vi "ImageGUI.vi"() -> ()   [LabVIEW 2017]
uses:
  <vilib>/Utility/miscctls.llb/LVPoint32TypeDef.ctl
  <vilib>/userdefined/High Color/IMAQdx.ctl
  <vilib>/vision/driver/NI_Vision_Acquisition_Software.lvlib
  <vilib>/vision/NI_Vision_Development_Module.lvlib
panel:
  out "Standard Variation":sgl
  out "SnapshotObjects":T1(array[cluster]) {"Aspect Ratio" format="%.2f"; "Orientation" format="%.2f"; "Area" format="%.2f"; "Object Center"."Y" format="%.2f"; "Object Center"."X" format="%.2f"}
  in  "SnapshotObjectsSettings":T2={"Objects"=0, "Threshold"=20, "Reject Border"=TRUE, "Fill Holes"=TRUE, "Min Object Size"=TRUE, "Min Size"=10, "Max Object Size"=FALSE, "Max Size"=100, "Show Search Area"=FALSE, "Show Center"=FALSE, "Show Bounding Box"=TRUE} {"Objects" items=["Bright Objects", "Dark Objects"]; "Threshold" min=1 max=999999999 step=1; "Max Size" min=1 max=999999999 step=1; "Min Size" min=1 max=999999999 step=1}
  in  "executed?":bool=TRUE
  out "result_from_daq":string
  in  "cmd2daq":string
  out "Difference Objects":T1(array[cluster]) {"Aspect Ratio" format="%.2f"; "Orientation" format="%.2f"; "Area" format="%.2f"; "Object Center"."Y" format="%.2f"; "Object Center"."X" format="%.2f"}
  in  "Buffer Length":i32=50
  in  "Settings":T2={"Objects"=0, "Threshold"=200, "Reject Border"=FALSE, "Fill Holes"=FALSE, "Min Object Size"=TRUE, "Min Size"=500, "Max Object Size"=TRUE, "Max Size"=800, "Show Search Area"=FALSE, "Show Center"=TRUE, "Show Bounding Box"=TRUE} {"Objects" items=["Bright Objects", "Dark Objects"]; "Threshold" min=1 max=999999999 step=1; "Max Size" min=1 max=999999999 step=1; "Min Size" min=1 max=999999999 step=1}
  in  "upper limit aspect ratio":sgl=1.4
  in  "lower limit aspect ratio":sgl=0.7
  out "#FOV":i32
  out "#tethers":i32
  out "#tasklist":i32
  out "status:":string="wait for tasklist to be finished"
  in  "number of tasklists to run":u32=2
  out "information of tethers":T3(array[cluster])
  in  "save all tether coordinates":bool
  in  "start automatic measurement":bool
  in  "Display Image":u16(ring) items=["Capture", "Capture with tracking", "Difference", "Objects"]
  in  "Find Objects":bool
  in  "Refresh timout (ms)":i32=100
  out "Last sent value (mm)":dbl[](array[numeric])
  in  "Zoom":dbl(slide) scale=1.0..4.0
  out "ROI":T4
  in  "Pixel Calibration":cluster{"X (nm/px)":dbl, "Y (nm/px)":dbl}={"X (nm/px)"=58.6, "Y (nm/px)"=58.6}
  out "RelativeClick":cluster{"X":i32, "Y":i32}
  in  "TrapCenter":cluster{"X":i32, "Y":i32}={"X"=982, "Y"=593}
  out "Coords":T5
  out "Image":T6(plugin-control)
  in  "stop":bool
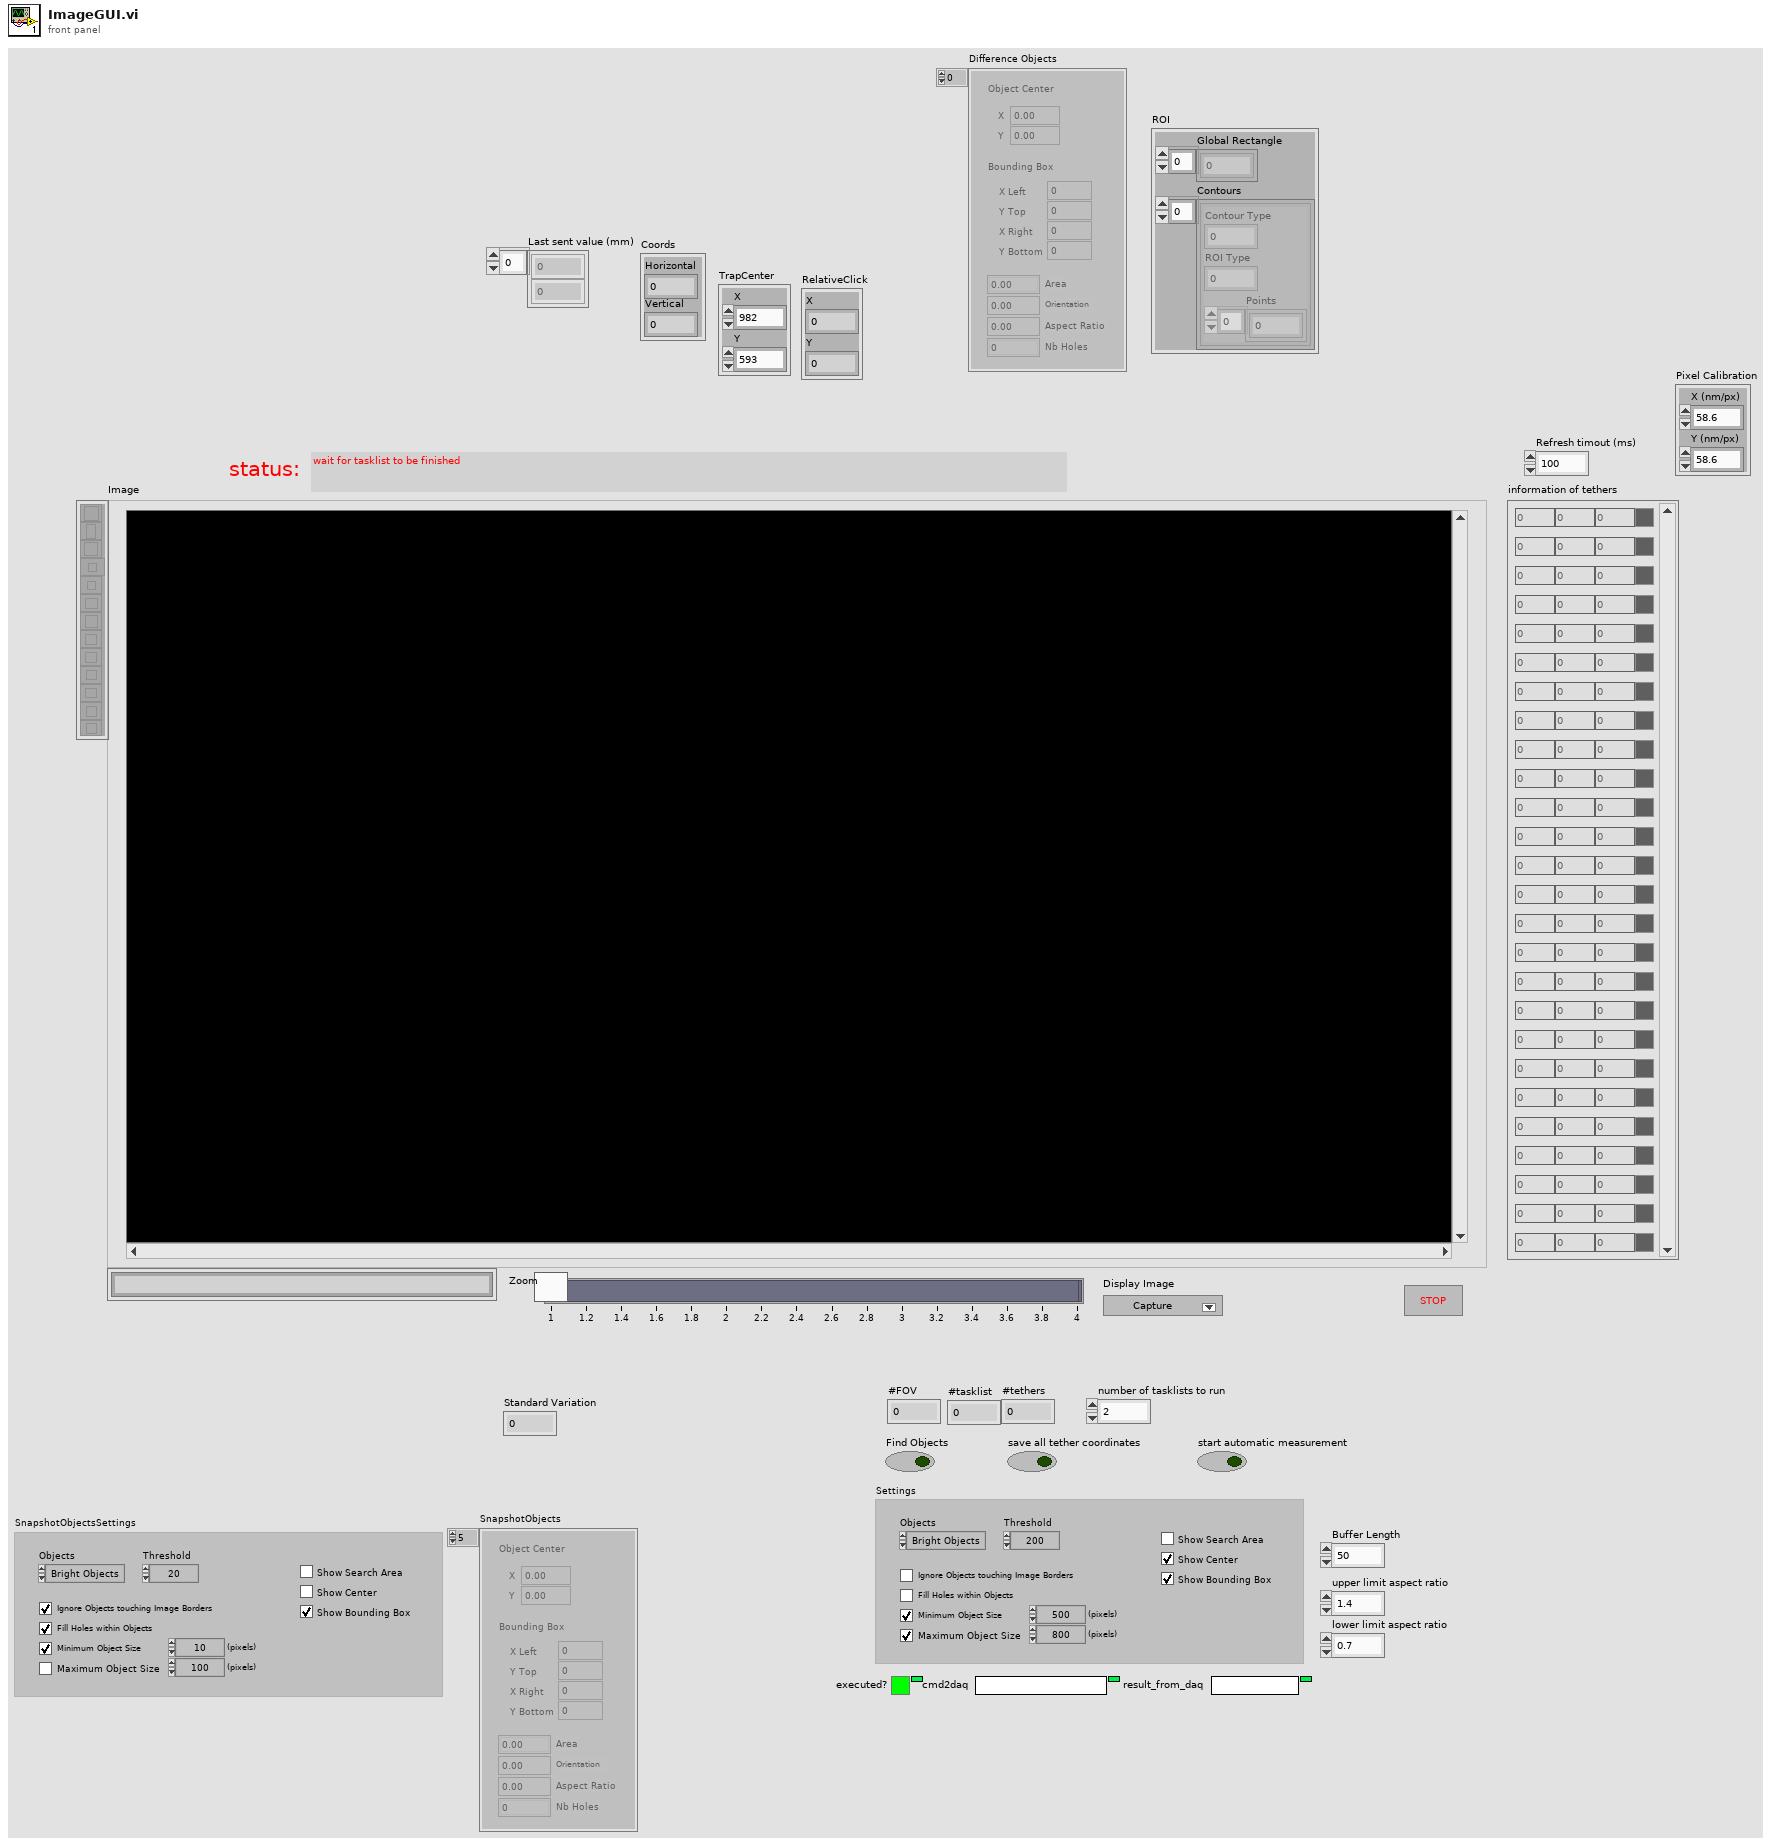
[diagram p1: front panel]
types:
  T1 = cluster{"Object Center":cluster{"X":sgl, "Y":sgl}, "Bounding Box":cluster{"X Left":i32, "Y Top":i32, "X Right":i32, "Y Bottom":i32}, "Area":sgl, "Orientation":sgl, "Aspect Ratio":sgl, "Nb Holes":i32}[]
  T2 = cluster{"Objects":u16, "Threshold":i32, "Reject Border":bool, "Fill Holes":bool, "Min Object Size":bool, "Min Size":i32, "Max Object Size":bool, "Max Size":i32, "Show Search Area":bool, "Show Center":bool, "Show Bounding Box":bool}
  T3 = cluster{"index":i32, "X":dbl, "Y":dbl, "good?":bool}[]
  T4 = cluster{"Global Rectangle":i32[], "Contours":cluster{"Contour Type":u32, "ROI Type":u32, "Points":i32[]}[]}
  T5 = typedef "LVPoint32TypeDef.ctl" = cluster{"Horizontal":i32, "Vertical":i32}
  T6 = typedef "IMAQ Image.ctl" = refnum<image>
  T7 = typedef "Image Type" = u32
  T8 = typedef "IMAQdx.ctl" = refnum<k21>
  T9 = cluster{"Contour Type":u32, "ROI Type":u32, "Points":i32[]}
  T10 = cluster{"Shift":bool, "Ctrl":bool, "Alt":bool, "Cmd":bool, "Opt":bool}
  T11 = cluster{"Contour Type":u32, "ROI Type":u32, "Points":i32[]}[]
  T12 = cluster{"Mean Value":sgl, "Standard Variation":sgl, "Minimal Value":sgl, "Maximal Value":sgl, "Area (calibrated)":sgl, "Area (pixels)":u32, "%":sgl, "Calibration Valid":bool}
  T13 = cluster{"X Left":i32, "Y Top":i32, "X Right":i32, "Y Bottom":i32}
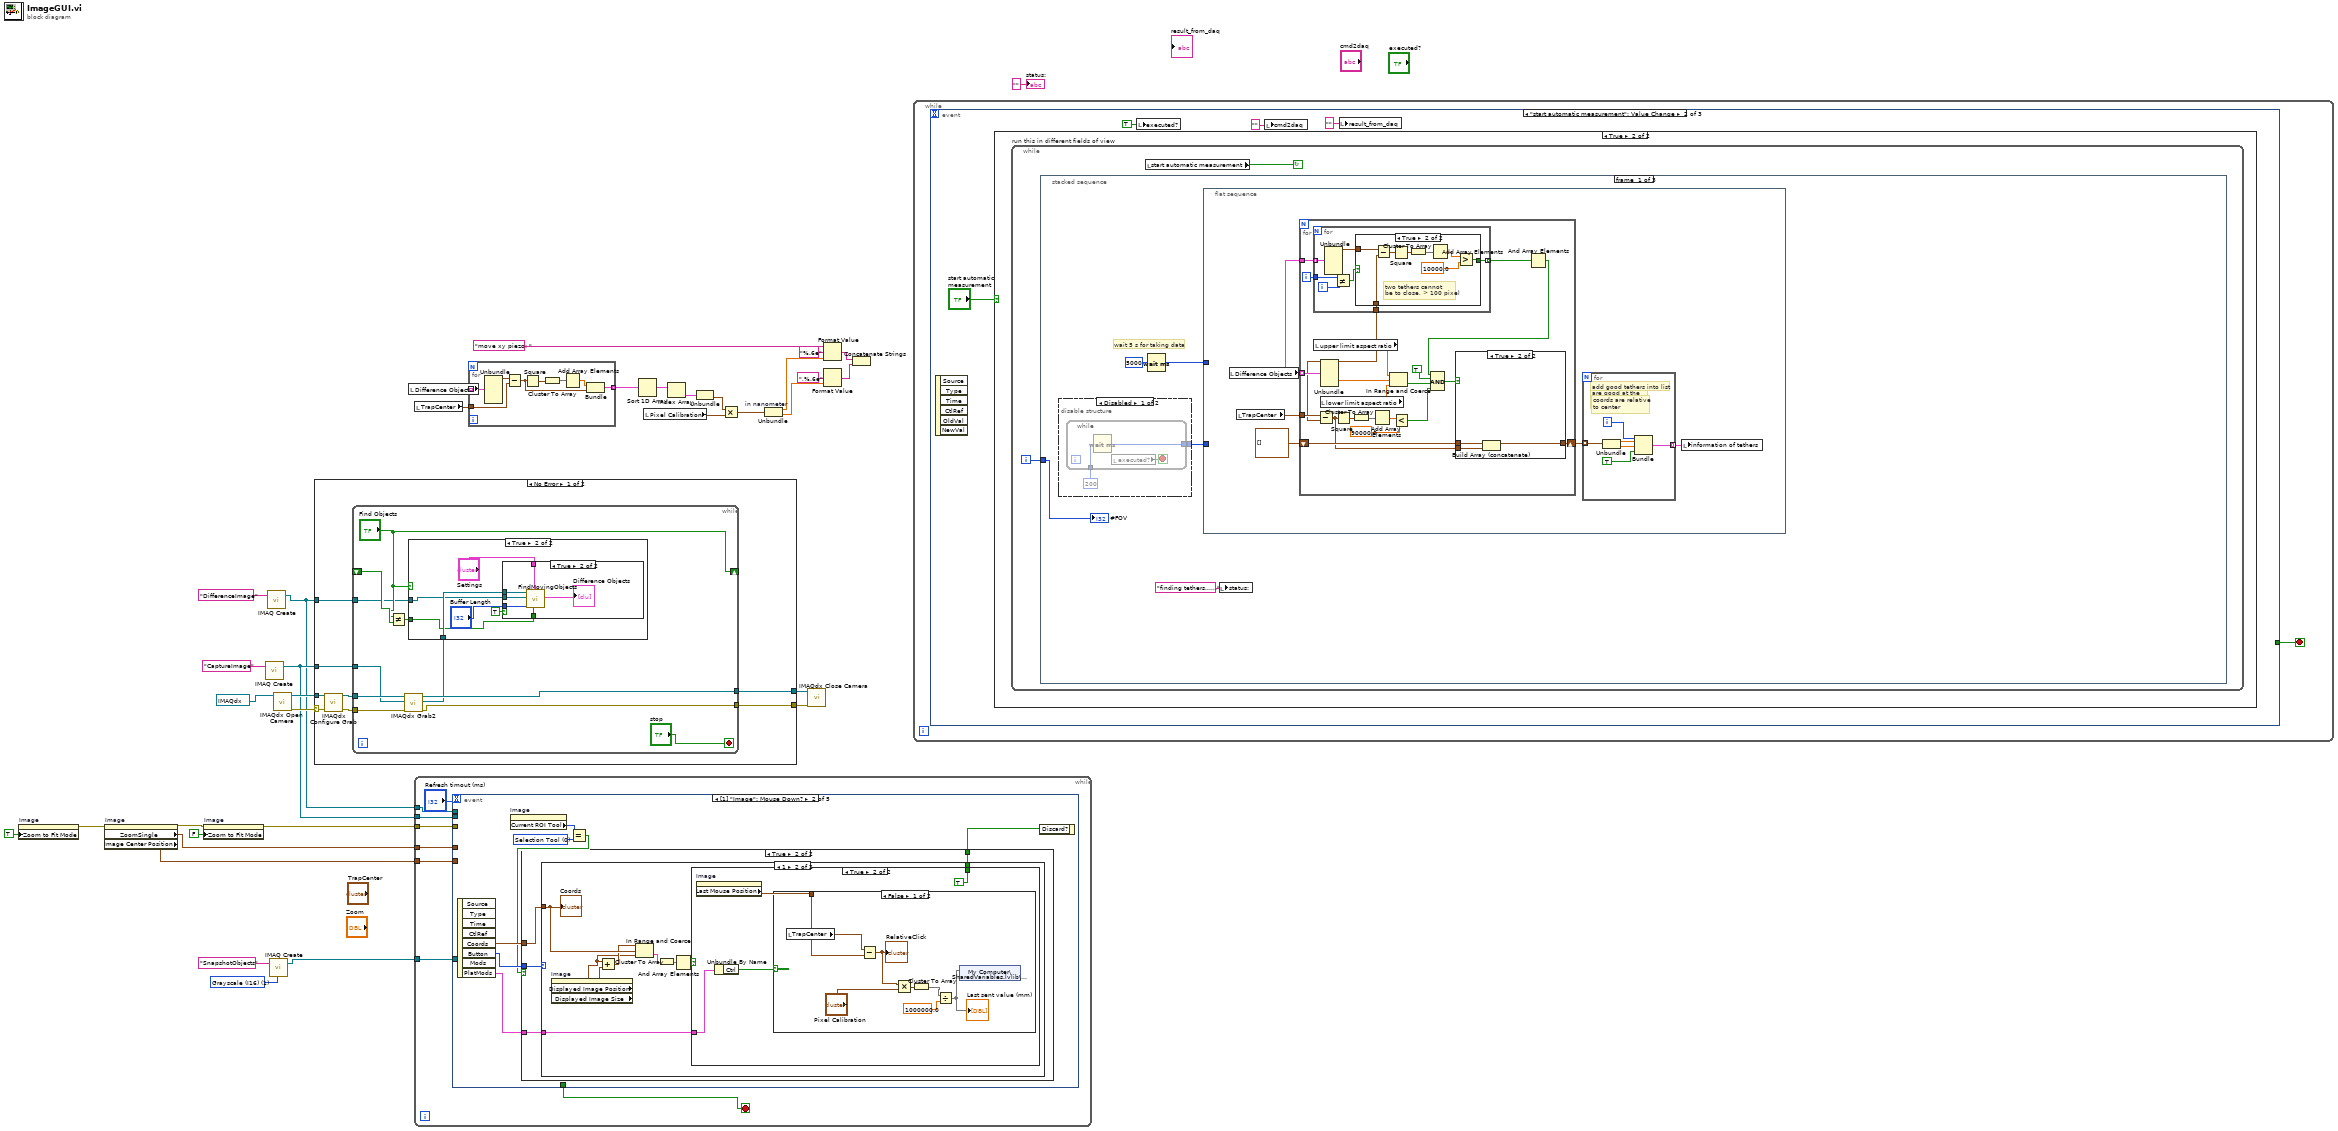
[diagram p0: block diagram]
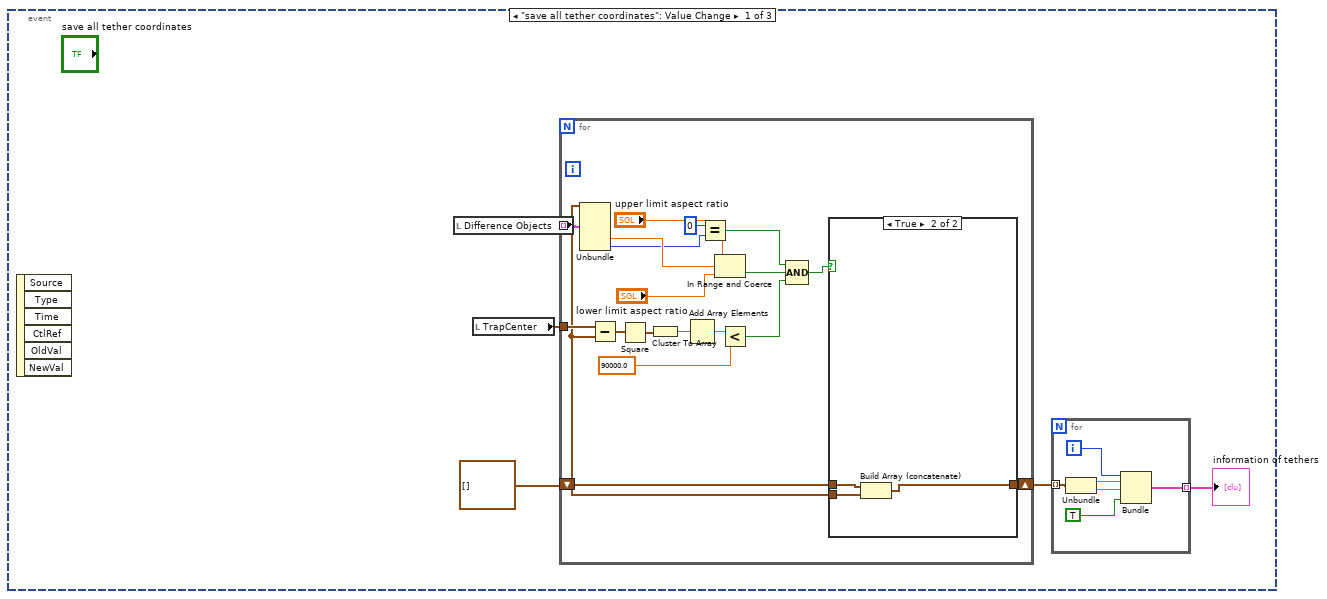
[diagram p2: hidden frame]
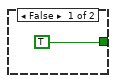
[diagram p6: hidden frame]
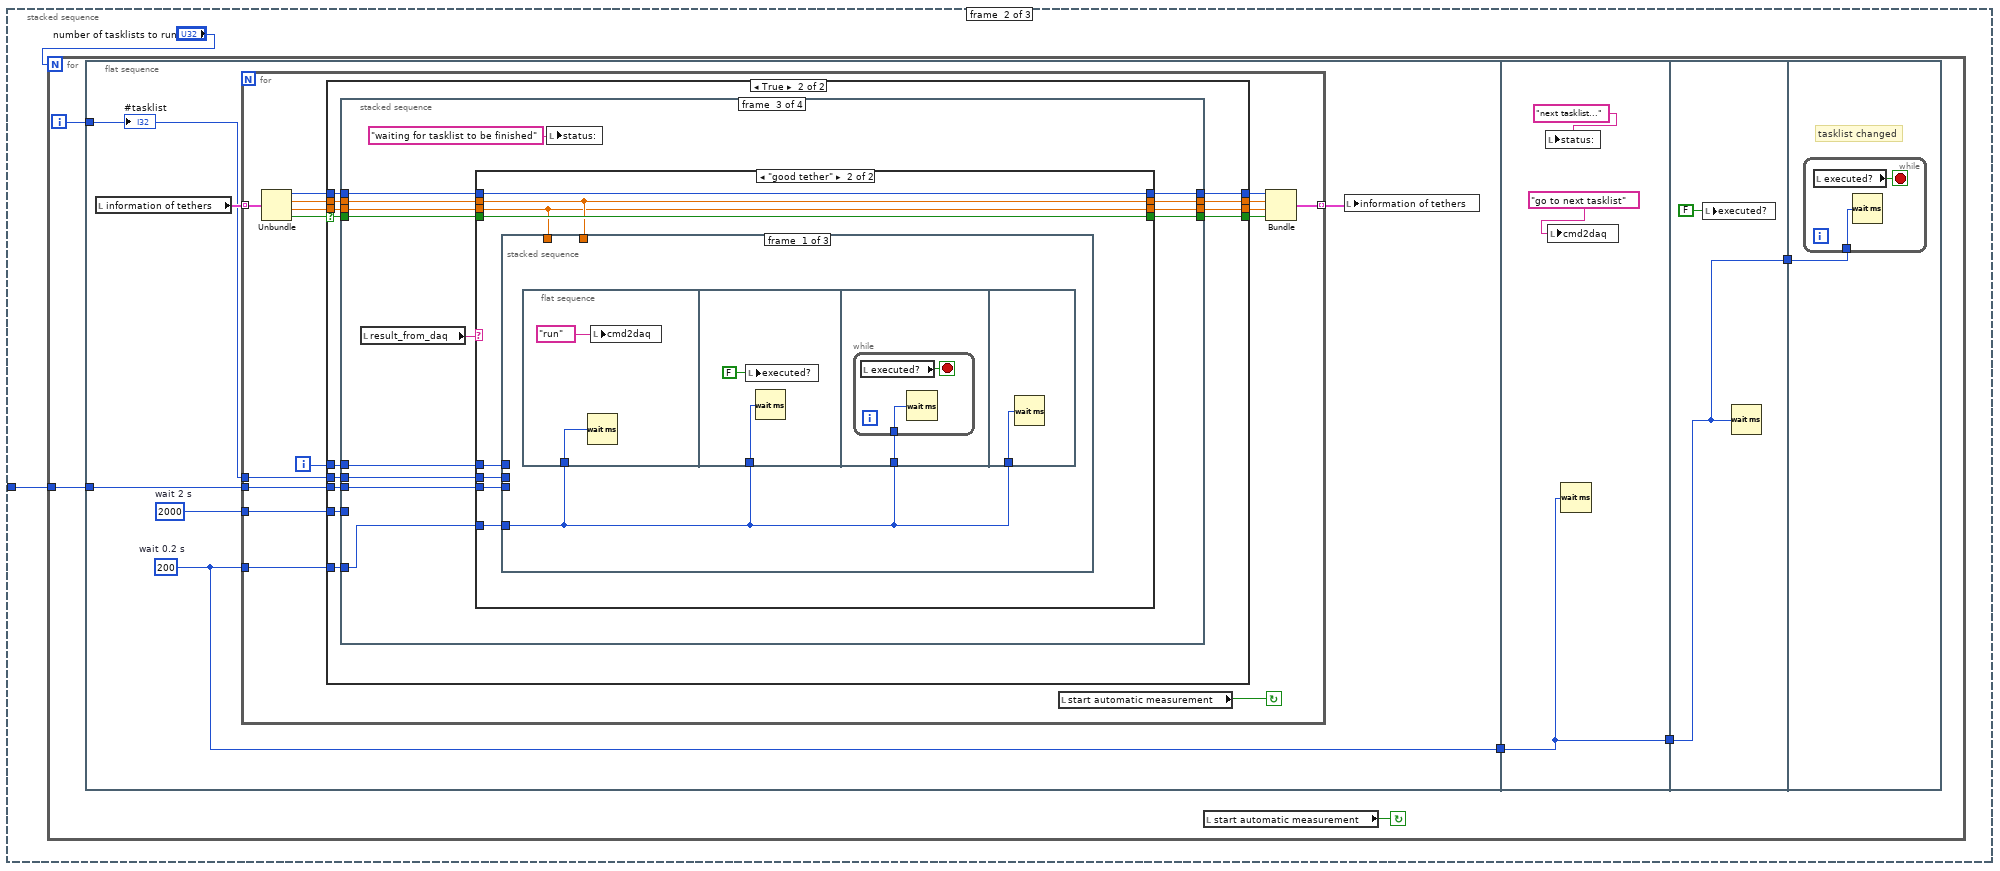
[diagram p8: hidden frame]
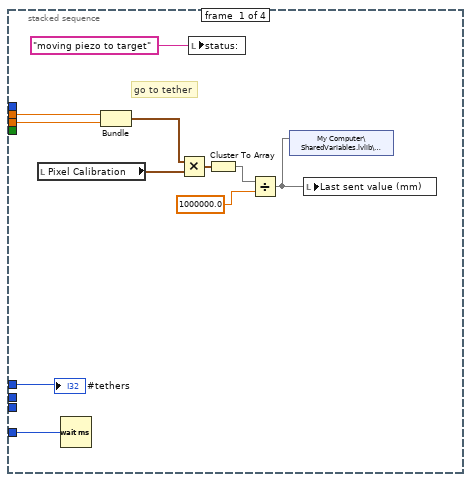
[diagram p10: hidden frame]
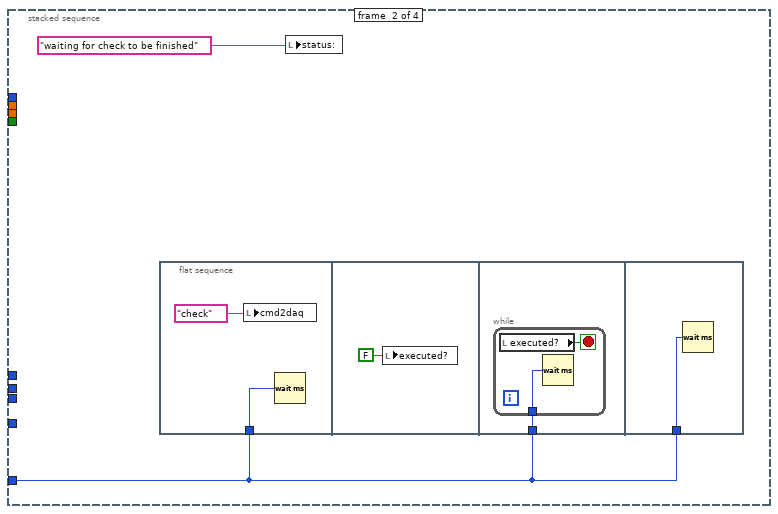
[diagram p11: hidden frame]
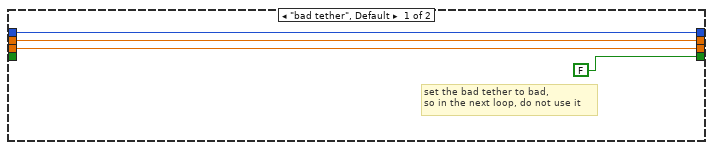
[diagram p12: hidden frame]
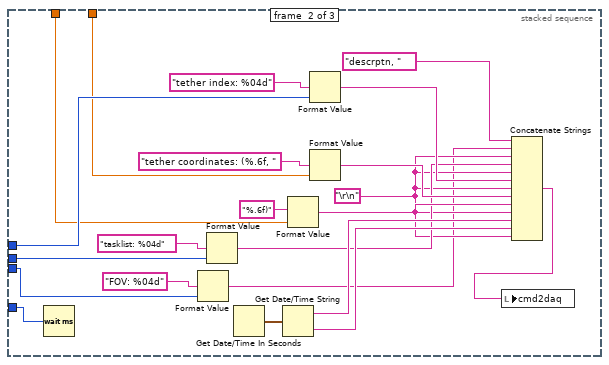
[diagram p13: hidden frame]
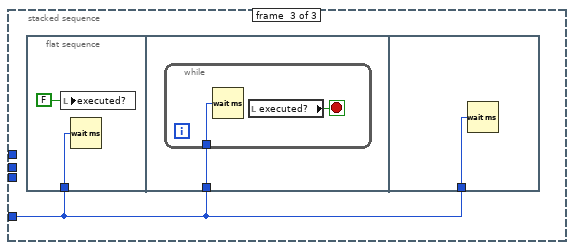
[diagram p14: hidden frame]
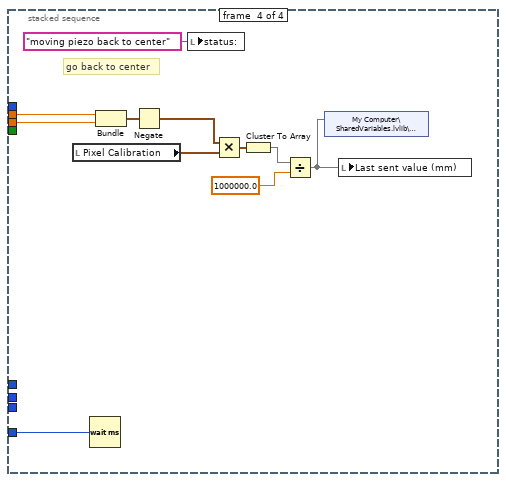
[diagram p15: hidden frame]
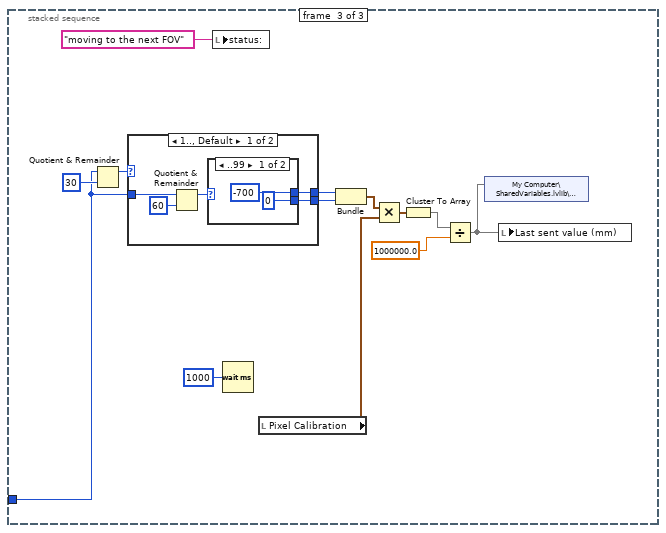
[diagram p16: hidden frame]
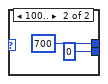
[diagram p17: hidden frame]
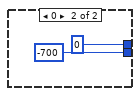
[diagram p18: hidden frame]
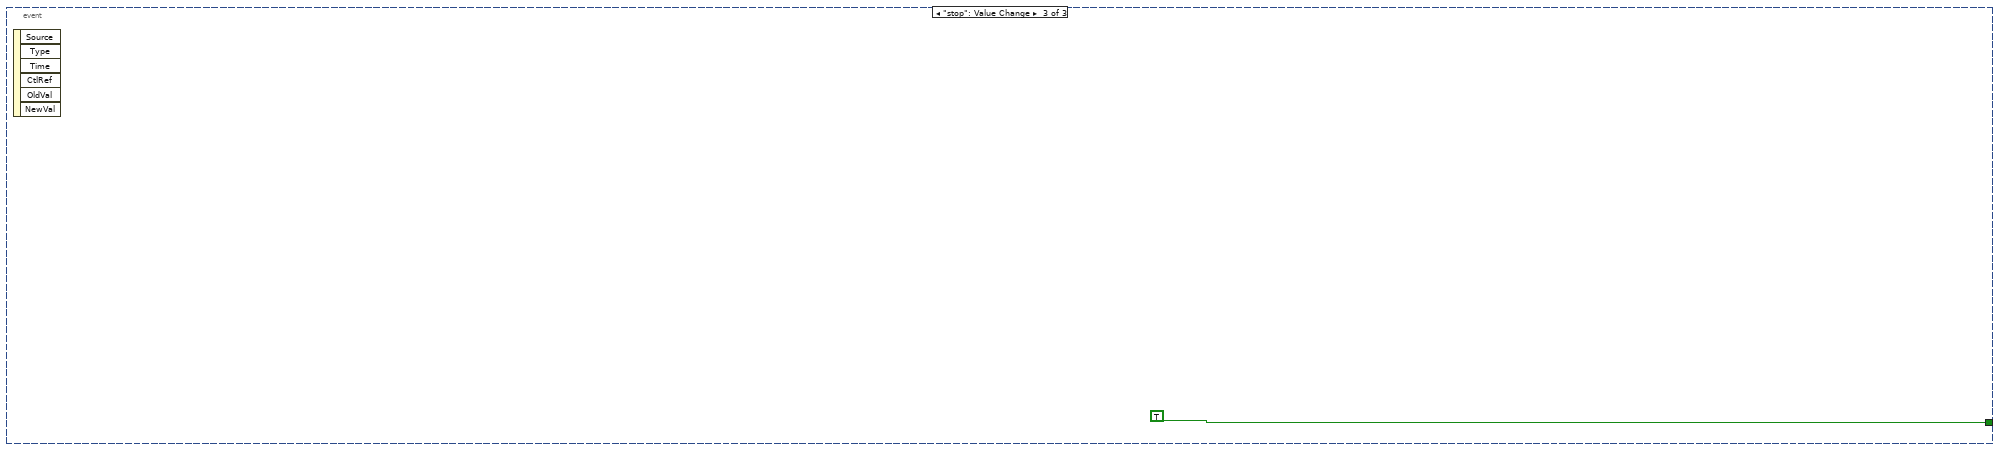
[diagram p19: hidden frame]
diagram:
  w1 = T7 1 items=["Grayscale (U8)", "Grayscale (I16)", "Grayscale (SGL)", "Complex (CSG)", "RGB (U32)", "HSL (U32)", "RGB (U64)", "Grayscale (U16)"] ("Image Type")
  n1 = property on="Image" class="ImageControl"("Zoom to Fit Mode"=TRUE) -> (error out=w32:errorcluster)  [unwired: 2 in, 1 out]
  n2 = property on="Image" class="ImageControl"(error in=w32) -> (error out=w31:errorcluster, "ZoomSingle"=w28:cluster{"X":sgl, "Y":sgl}, "Image Center Position"=w27:cluster{"X":u32, "Y":u32})  [unwired: 1 in, 1 out]
  n3 = property on="Image" class="ImageControl"(error in=w31, "Zoom to Fit Mode"=FALSE) -> (error out=w29:errorcluster)  [unwired: 1 in, 1 out]
  n4 = call "IMAQ Create"("Image Name"="CaptureImage") -> ("New Image"=w22:T6)  [unwired: 4 in, 1 out]
  n5 = call "IMAQ Create"("Image Name"="DifferenceImage") -> ("New Image"=w20:T6)  [unwired: 4 in, 1 out]
  n6 = call "IMAQ Create"("Image Name"="SnapshotObjects", "Image Type"=w1) -> ("New Image"=w2:T6)  [unwired: 3 in, 1 out]
  n7 = call <vilib>:"IMAQdx Open Camera.vi"("Session In"=T8 "cam0") -> ("error out"=w26:errorcluster, "Session Out"=w34:T8)  [unwired: 9 in]
  n8 = case shown="No Error" w26 {
    selector: w26 -> [w40 w68]
    tunnel: w34 -> [w43 w67]
    tunnel: [w39 w68] -> w25
    tunnel: [w38 w67] -> w24
    tunnel: w22 -> [w37 _]
    tunnel: w20 -> [w36 _]
    frame No Error {
      n9 = call <vilib>:"IMAQdx Configure Grab.vi"("error in"=w40, "Session In"=w43) -> ("error out"=w41:errorcluster, "Session Out"=w42:T8)  [unwired: 8 in]
      n10 = while {
        tunnel: w42 -> [w54]
        tunnel: w41 -> [w53]
        tunnel: [w51] -> w39
        tunnel: [w50] -> w38
        tunnel: w37 -> [w49]
        tunnel: w36 -> [w44]
        shift-right: ["Find Objects"] -> _
        shift-left: _ -> [w47]
        stop <- "stop" stop-if-true
        n11 = Not Equal?(x="Find Objects", y=w47) -> (x != y?=w45:bool)
        n12 = call <vilib>:"IMAQdx Grab2.vi"("error in"=w53, "Image In"=w49, "Session In"=w54) -> ("error out"=w51:errorcluster, "Image Out"=w48:T6, "Session Out"=w50:T8)  [unwired: 5 in, 1 out]
        n13 = case shown="True" "Find Objects" {
          tunnel: w48 -> [_ w60]
          tunnel: w44 -> [_ w59]
          tunnel: w45 -> [_ w56]
          frame False {
          }
          frame True {
            n14 = case shown="True" TRUE {
              tunnel: w60 -> [_ w61]
              tunnel: w59 -> [_ w66]
              tunnel: "Buffer Length" -> [_ w65]
              tunnel: "Settings" -> [_ w64]
              tunnel: w56 -> [_ w63]
              frame False {
              }
              frame True {
                n15 = call "FindMovingObjects.vi"("Initialize?"=w63, "Settings"=w64, "Buffer Length"=w65, "Image Dst"=w66, "Image Src"=w61) -> ("Objects"=→"Difference Objects":T1)  [unwired: 5 in, 1 out]
              }
            }
          }
        }
      }
    }
    frame Error {
    }
  }
  n16 = local read "Difference Objects"() -> (w17:T1)
  n17 = local read "TrapCenter"() -> (w18:cluster{"X":i32, "Y":i32})
  n18 = while {
    tunnel: w29 -> [w75]
    tunnel: w28 -> [w74]
    tunnel: w27 -> [w73]
    tunnel: w22 -> [w71]
    tunnel: w20 -> [w70]
    tunnel: w2 -> [w69]
    stop <- w76 stop-if-true
    n19 = event shown="[1] \"Image\": Mouse Down?" {
      selector: _ -> [_ _ _ _ _]
      dyn-events: _ -> [_ _ _ _ _]
      timeout: "Refresh timout (ms)" -> [_ _ _ _ _]
      tunnel: [w77 _ _ _ _] -> w76
      tunnel: w75 -> [_ _ _ _ _]
      tunnel: w74 -> [_ _ _ w169 _]
      tunnel: w73 -> [_ _ _ w166 _]
      tunnel: w71 -> [_ _ w127 _ _]
      tunnel: w70 -> [_ _ w130 _ _]
      tunnel: w69 -> [_ _ w129 _ _]
      event "stop": Value Change {
        n20 = event-data() -> ("NewVal"=w77:bool)  [unwired: 1 in, 5 out]
      }
      event "Image": Mouse Down? {
        w81 = u32 0 items=["Zoom Tool"=8, "Selection Tool"=0, "Pan Tool"=9, "Point Tool"=1, "Line Tool"=2, "Rectangle Tool"=3, "Rotated Rectangle Tool"=12, "Polyline Tool"=10, "Polygon Tool"=5, "Freehand Tool"=11, "Closed Freehand Tool"=6, "Ellipse Tool"=4, "Annulus Tool"=7] ("Current ROI Tool")
        n21 = event-data() -> ("Coords"=w84:T5, "Button"=w83:u16, "PlatMods"=w82:T10)  [unwired: 1 in, 5 out]
        n22 = property on="Image" class="ImageControl"() -> ("Current ROI Tool"=w80:u32)  [unwired: 2 in, 2 out]
        n23 = Equal?(x=w80, y=w81) -> (x = y?=w79:bool)
        n24 = case shown="True" w79 {
          tunnel: w84 -> [_ w88]
          tunnel: w83 -> [_ w87]
          tunnel: w82 -> [_ w86]
          tunnel: [_ w85] -> w78
          frame False {
          }
          frame True {
            n25 = case shown="1" w87 {
              tunnel: w88 -> [_ w97]
              tunnel: w86 -> [_ w90]
              tunnel: [_ w89] -> w85
              frame 0, Default {
              }
              frame 1 {
                n26 = property on="Image" class="ImageControl"() -> ("Displayed Image Position"=w92:cluster{"Left":i32, "Top":i32}, "Displayed Image Size"=w91:cluster{"Width":u32, "Height":u32})  [unwired: 2 in, 2 out]
                n27 = Add(x=w92, y=w91) -> (x+y=w96:cluster{u32, u32})
                n28 = In Range and Coerce(upper limit=w96, x=w97, lower limit=w92) -> (In Range?=w95:cluster{"Horizontal":bool, "Vertical":bool})  [unwired: 1 out]
                n29 = Cluster To Array(cluster=w95) -> (array=w94:bool[])
                n30 = And Array Elements(Boolean array=w94) -> (logical AND=w93:bool)
                n31 = case shown="True" w93 {
                  tunnel: w90 -> [_ w101]
                  tunnel: [_ TRUE ("Discard?")] -> w89
                  frame False {
                  }
                  frame True {
                    n32 = property on="Image" class="ImageControl"() -> ("Last Mouse Position"=w99:cluster{"X":i32, "Y":i32})  [unwired: 2 in, 2 out]
                    n33 = Unbundle By Name(w101) -> ("Ctrl"=w100:bool)
                    n34 = case shown="False" w100 {
                      tunnel: w99 -> [w109 w122]
                      frame False {
                        n35 = local read "TrapCenter"() -> (w108:cluster{"X":i32, "Y":i32})
                        n36 = Subtract(x=w108, y=w109) -> (x-y=w107:cluster{"X":i32, "Y":i32})
                        "RelativeClick" <- w107
                        n37 = Multiply(x=w107, y="Pixel Calibration") -> (x*y=w105:cluster{dbl, dbl})
                        n38 = Cluster To Array(cluster=w105) -> (array=w104:dbl[])
                        n39 = Divide(x=w104, y=1000000.0) -> (x/y=w102:dbl[])
                        "Last sent value (mm)" <- w102
                        n40 = shared-variable "My Computer\\SharedVariables.lvlib\\ImageClick"(w102) -> ()  [unwired: 1 in, 1 out]
                      }
                      frame True {
                        w110 = u32 1 ("Contour Type")
                        n41 = property on="TrapCenter" class="Clust (strict)"("Val(Sgnl)"=w122) -> ()  [unwired: 2 in, 2 out]
                        n42 = Add(x=w122, y=w110) -> (x+y=w120:cluster{"X":u32, "Y":u32})
                        n43 = Subtract(x=w122, y=w110) -> (x-y=w121:cluster{"X":u32, "Y":u32})
                        n44 = Cluster To Array(cluster=w121) -> (array=w119:u32[])
                        n45 = Cluster To Array(cluster=w120) -> (array=w118:u32[])
                        n46 = Build Array (concatenate)(w119, w118) -> (w113:u32[])
                        n47 = Bundle By Name(cluster=T9 {"Contour Type"=0, "ROI Type"=0, "Points"=[]}, "Contour Type"=u32 0, "ROI Type"=w110, "Points"=w113) -> (w115:T9)
                        n48 = Build Array(w115) -> (w114:T11)
                        n49 = Bundle By Name(cluster=T4 {"Global Rectangle"=[], "Contours"=[]} ("ROI"), "Global Rectangle"=w113, "Contours"=w114) -> (w112:T4)
                        "ROI" <- w112
                        n50 = property on="Image" class="ImageControl"("ROI"=w112) -> ()  [unwired: 2 in, 2 out]
                      }
                    }
                  }
                }
                "Coords" <- w97
              }
            }
          }
        }
        n51 = event-data("Discard?"=w78) -> ()  [unwired: 1 in, 1 out]
      }
      event Timeout {
        n52 = event-data() -> ()  [unwired: 1 in, 3 out]
        n53 = call "IMAQ GetImageSize"("Image"=w127) -> ("Y Resolution"=w126:i32)  [unwired: 3 in, 2 out]
        n54 = Greater Than 0?(x=w126) -> (x > 0?=w125:bool)
        n55 = case shown="True" w125 {
          tunnel: w129 -> [w132 w147]
          tunnel: [w132 w139] -> w128
          tunnel: w127 -> [_ w141]
          tunnel: [_ w133] -> w124
          frame False {
          }
          frame True {
            n56 = call "IMAQ Copy"("Image Dst"=w147, "Image Src"=w141) -> ("Image Dst Out"=w146:T6)  [unwired: 4 in, 1 out]
            n57 = call "IMAQ Quantify 2"("Image"=w146) -> ("Global Report"=w145:T12)  [unwired: 8 in, 2 out]
            n58 = Unbundle By Name(w145) -> ("Mean Value"=w144:sgl, "Standard Variation"=→"Standard Variation":sgl)
            n59 = call "IMAQ Absolute Difference"("Image Src A"=w146, "Constant"=w144) -> ("Image Dst Out"=w143:T6)  [unwired: 5 in, 1 out]
            n60 = Unbundle By Name("SnapshotObjectsSettings") -> ("Threshold"=w136:i32)
            n61 = call "IMAQ Count Objects 2"("Settings"="SnapshotObjectsSettings", "Image"=w143) -> ("Image Out"=w140:T6, "Objects"=w133:T1)  [unwired: 5 in, 3 out]
            "SnapshotObjects" <- w133
            n62 = Bundle("Threshold"=w136, inf) -> (w135:cluster{"Threshold":i32, dbl})  [unwired: 1 out]
            n63 = call "IMAQ Threshold"("Replace Value"=sgl 255.0, "Range"=w135, "Image Src"=w140) -> ("Image Dst Out"=w139:T6)  [unwired: 7 in, 1 out]
          }
        }
        n64 = case shown="3" "Display Image" {
          tunnel: w127 -> [w148 w149 _ _]
          tunnel: [w148 w150 w164 w165] -> w123
          tunnel: w130 -> [_ _ w164 _]
          tunnel: w128 -> [_ _ _ w165]
          tunnel: w124 -> [_ w151 _ _]
          frame 0, Default {
          }
          frame 1 {
            n65 = local read "Difference Objects"() -> (w152:T1)
            n66 = for {
              tunnel: w152 -> [w160] mode=indexing
              tunnel: w149 -> [w163]
              tunnel: [w159] -> _
              n67 = Unbundle By Name(w160) -> ("Bounding Box"=w162:T13)
              n68 = call "IMAQ Overlay Rectangle"("Color"=u32 16711680, "Rectangle"=w162, "Image"=w163) -> ("error out"=w159:errorcluster)  [unwired: 7 in, 1 out]
            }
            n69 = for {
              tunnel: w151 -> [w158] mode=indexing
              tunnel: [w155] -> w150
              tunnel: [w154] -> _
              tunnel: w149 -> [w153]
              n70 = Unbundle By Name(w158) -> ("Bounding Box"=w157:T13)
              n71 = call "IMAQ Overlay Rectangle"("Color"=u32 6618880, "Rectangle"=w157, "Image"=w153) -> ("error out"=w154:errorcluster, "Image Out"=w155:T6)  [unwired: 7 in]
            }
          }
          frame 2 {
          }
          frame 3 {
          }
        }
        "Image" <- w123
      }
      event "Zoom": Value Change {
        n72 = event-data() -> ("NewVal"=w168:dbl)  [unwired: 1 in, 5 out]
        n73 = Multiply(x=w169, y=w168) -> (x*y=w167:cluster{"X":dbl, "Y":dbl})
        n74 = property on="Image" class="ImageControl"("ZoomSingle"=w167, "Image Center Position"=w166) -> ()  [unwired: 2 in, 2 out]
      }
      event "TrapCenter": Value Change {
        n75 = event-data() -> ()  [unwired: 1 in, 6 out]
      }
    }
  }
  n76 = for {
    tunnel: w17 -> [w177] mode=indexing
    tunnel: w18 -> [w173]
    tunnel: [w170] -> w16 mode=indexing
    n77 = Unbundle(w177) -> ("Object Center"=w174:cluster{"X":sgl, "Y":sgl})  [unwired: 5 out]
    n78 = Subtract(x=w174, y=w173) -> (x-y=w171:cluster{"X":sgl, "Y":sgl})
    n79 = Square(x=w171) -> (x^2=w176:cluster{"X":sgl, "Y":sgl})
    n80 = Cluster To Array(cluster=w176) -> (array=w175:sgl[])
    n81 = Add Array Elements(numeric array=w175) -> (sum=w172:sgl)
    n82 = Bundle("X"=w172, w171) -> (w170:cluster{"X":sgl, cluster{"X":sgl, "Y":sgl}})  [unwired: 1 in]
  }
  n83 = Sort 1D Array(array=w16) -> (sorted array=w15:cluster{"X":sgl, cluster{"X":sgl, "Y":sgl}}[])
  n84 = local read "Pixel Calibration"() -> (w12:cluster{"X (nm/px)":dbl, "Y (nm/px)":dbl})
  n85 = Index Array(array=w15) -> (element=w14:cluster{"X":sgl, cluster{"X":sgl, "Y":sgl}})  [unwired: 1 in]
  n86 = Unbundle(w14) -> (w13:cluster{"X":sgl, "Y":sgl})  [unwired: 1 out]
  n87 = Multiply(x=w13, y=w12) -> (x*y=w11:cluster{dbl, dbl})
  n88 = Unbundle "in nanometer"(w11) -> (w9:dbl, w6:dbl)
  n89 = call <vilib>:"IMAQdx Close Camera.vi"("error in"=w25, "Session In"=w24) -> ()  [unwired: 9 in, 1 out]
  n90 = Format Value(string ("")="move xy piezo: ", format string="%.6e", value (0)=w9) -> (output string=w5:string)
  n91 = Format Value(format string=",%.6e", value (0)=w6) -> (output string=w4:string)  [unwired: 1 in]
  n92 = Concatenate Strings(w5, w4) -> ()  [unwired: 1 out]
  n93 = while {
    stop <- w178 stop-if-true
    n94 = event shown="[1] \"start automatic measurement\": Value Change" {
      selector: _ -> [_ _ _]
      dyn-events: _ -> [_ _ _]
      timeout: _ -> [_ _ _]
      tunnel: [_ _ TRUE] -> w178
      event "save all tether coordinates": Value Change {
        n95 = event-data() -> ()  [unwired: 1 in, 6 out]
        n96 = local read "Difference Objects"() -> (w182:T1)
        n97 = local read "TrapCenter"() -> (w181:cluster{"X":i32, "Y":i32})
        n98 = for {
          tunnel: w182 -> [w201] mode=indexing
          shift-right: [w202] -> w180
          shift-left: cluster{"X":sgl, "Y":sgl}[] [] -> [w203]
          tunnel: w181 -> [w200]
          n99 = Unbundle(w201) -> ("Object Center"=w199:cluster{"X":sgl, "Y":sgl}, "Aspect Ratio"=w208:sgl, "Nb Holes"=w207:i32)  [unwired: 3 out]
          n100 = Subtract(x=w200, y=w199) -> (x-y=w198:cluster{"X":sgl, "Y":sgl})
          n101 = Square(x=w198) -> (x^2=w197:cluster{"X":sgl, "Y":sgl})
          n102 = Cluster To Array(cluster=w197) -> (array=w196:sgl[])
          n103 = Add Array Elements(numeric array=w196) -> (sum=w195:sgl)
          n104 = Equal?(x=0, y=w207) -> (x = y?=w193:bool)
          n105 = In Range and Coerce(upper limit="upper limit aspect ratio", x=w208, lower limit="lower limit aspect ratio") -> (In Range?=w192:bool)  [unwired: 1 out]
          n106 = Less?(x=w195, y=sgl 90000.0) -> (x < y?=w191:bool)
          n107 = Compound Arithmetic op=AND(w193, w192, w191) -> (w190:bool)
          n108 = case shown="True" w190 {
            tunnel: w203 -> [w209 w212]
            tunnel: [w209 w211] -> w202
            tunnel: w199 -> [_ w210]
            frame False {
            }
            frame True {
              n109 = Build Array (concatenate)(w212, w210) -> (w211:cluster{"X":sgl, "Y":sgl}[])
            }
          }
        }
        n110 = for {
          tunnel: w180 -> [w187] mode=indexing
          tunnel: [w184] -> w179 mode=indexing
          i -> [w185]
          n111 = Unbundle(w187) -> ("X"=w188:sgl, "Y"=w186:sgl)
          n112 = Bundle(w185, "X"=w188, "Y"=w186, TRUE) -> (w184:cluster{i32, "X":sgl, "Y":sgl, bool})  [unwired: 1 in]
        }
        "information of tethers" <- w179
      }
      event "start automatic measurement": Value Change {
        n113 = event-data() -> ()  [unwired: 1 in, 6 out]
        n114 = case shown="True" "start automatic measurement" {
          frame False {
          }
          frame True {
            n115 = while "run this in different fields of view" {
              i -> [w217]
              stop <- w218 continue-if-true
              n116 = stacked-sequence {
                tunnel: w217 -> [w219 w281 w431]
                frame #0 {
                  # "wait 5 s for taking data"
                  n117 = disable-structure shown="Disabled" {
                    disable-tunnel: [w224 _] -> w221
                    frame Disabled {
                      n118 = while {
                        tunnel: u32 200 ("wait 0.2 s") -> [w227]
                        tunnel: [w226] -> w224
                        stop <- w228 stop-if-true
                        n119 = Wait (ms)(milliseconds to wait=w227) -> (millisecond timer value=w226:u32)
                        n120 = local read "executed?"() -> (w228:bool)
                      }
                    }
                    frame Enabled {
                    }
                  }
                  n121 = Wait (ms)(milliseconds to wait=u32 5000) -> (millisecond timer value=w222:u32)
                  n122 = flat-sequence {
                    tunnel: w222 -> [_]
                    tunnel: w221 -> [_]
                    frame #0 {
                      n123 = local read "Difference Objects"() -> (w229:T1)
                      n124 = local read "TrapCenter"() -> (w233:cluster{"X":i32, "Y":i32})
                      n125 = for {
                        tunnel: w229 -> [w257] mode=indexing
                        shift-right: [w258] -> w232
                        shift-left: cluster{"X":sgl, "Y":sgl}[] [] -> [w259]
                        tunnel: w233 -> [w256]
                        tunnel: w229 -> [w244]
                        i -> [w242]
                        n126 = local read "upper limit aspect ratio"() -> (w247:sgl)
                        n127 = local read "lower limit aspect ratio"() -> (w248:sgl)
                        n128 = Unbundle(w257) -> ("Object Center"=w243:cluster{"X":sgl, "Y":sgl}, "Aspect Ratio"=w260:sgl)  [unwired: 4 out]
                        n129 = for {
                          tunnel: w244 -> [w267] mode=indexing
                          tunnel: w243 -> [w265]
                          tunnel: w242 -> [w263]
                          tunnel: [w261] -> w241 mode=indexing
                          i -> [w264]
                          n130 = Unbundle(w267) -> ("Object Center"=w266:cluster{"X":sgl, "Y":sgl})  [unwired: 5 out]
                          n131 = Not Equal?(x=w263, y=w264) -> (x != y?=w262:bool)
                          n132 = case shown="True" w262 {
                            tunnel: w266 -> [_ w273]
                            tunnel: w265 -> [_ w272]
                            tunnel: [TRUE w270] -> w261
                            frame False {
                            }
                            frame True {
                              # "two tethers cannot\nbe to close, > 100 pixel"
                              n133 = Subtract(x=w273, y=w272) -> (x-y=w274:cluster{"X":sgl, "Y":sgl})
                              n134 = Square(x=w274) -> (x^2=w276:cluster{"X":sgl, "Y":sgl})
                              n135 = Cluster To Array(cluster=w276) -> (array=w275:sgl[])
                              n136 = Add Array Elements(numeric array=w275) -> (sum=w271:sgl)
                              n137 = Greater?(x=w271, y=sgl 10000.0) -> (0:w270:bool)
                            }
                          }
                        }
                        n138 = Subtract(x=w256, y=w243) -> (x-y=w245:cluster{"X":sgl, "Y":sgl})
                        n139 = Square(x=w245) -> (x^2=w255:cluster{"X":sgl, "Y":sgl})
                        n140 = Cluster To Array(cluster=w255) -> (array=w254:sgl[])
                        n141 = Add Array Elements(numeric array=w254) -> (sum=w253:sgl)
                        n142 = In Range and Coerce(upper limit=w247, x=w260, lower limit=w248) -> (In Range?=w251:bool)  [unwired: 1 out]
                        n143 = Less?(x=w253, y=sgl 90000.0) -> (x < y?=w250:bool)
                        n144 = And Array Elements(Boolean array=w241) -> (logical AND=w240:bool)
                        n145 = Compound Arithmetic op=AND(w240, TRUE ("value"), w251, w250) -> (w249:bool)
                        n146 = case shown="True" w249 {
                          tunnel: w259 -> [w277 w280]
                          tunnel: [w277 w279] -> w258
                          tunnel: w245 -> [_ w278]
                          frame False {
                          }
                          frame True {
                            n147 = Build Array (concatenate)(w280, w278) -> (w279:cluster{"X":sgl, "Y":sgl}[])
                          }
                        }
                      }
                      n148 = for {
                        tunnel: w232 -> [w237] mode=indexing
                        tunnel: [w234] -> w231 mode=indexing
                        i -> [w235]
                        # "coords are relative\nto center"
                        # "add good tethers into list"
                        # "assume all tethers\nare good at the\nbeginning"
                        n149 = Unbundle(w237) -> ("X"=w238:sgl, "Y"=w236:sgl)
                        n150 = Bundle(w235, "X"=w238, "Y"=w236, TRUE) -> (w234:cluster{i32, "X":sgl, "Y":sgl, bool})  [unwired: 1 in]
                      }
                      n151 = local write "information of tethers"(w231) -> ()
                    }
                  }
                  n152 = local write "status:"("finding tethers......" ("status")) -> ()
                  "#FOV" <- w219
                }
                frame #1 {
                  n153 = for {
                    N: "number of tasklists to run" -> [_]
                    tunnel: w281 -> [w286]
                    i -> [w287]
                    stop <- w288 continue-if-true
                    n154 = flat-sequence {
                      tunnel: w287 -> [w292]
                      tunnel: w286 -> [w291]
                      tunnel: [w289] -> w285
                      tunnel: w285 -> [w424]
                      tunnel: [w424] -> w284
                      tunnel: w284 -> [w426]
                      tunnel: [w426] -> w283
                      tunnel: w283 -> [w428]
                      frame #0 {
                        w289 = u32 200  # wait 0.2 s
                        w293 = u32 2000  # wait 2 s
                        n155 = local read "information of tethers"() -> (w294:T3)
                        n156 = for {
                          tunnel: w294 -> [w310] mode=indexing
                          tunnel: w293 -> [w306]
                          tunnel: w289 -> [w303]
                          tunnel: w292 -> [w301]
                          tunnel: w291 -> [w300]
                          tunnel: [w295] -> w290 mode=indexing
                          i -> [w304]
                          stop <- w302 continue-if-true
                          n157 = Unbundle(w310) -> ("index"=w305:i32, "X"=w308:dbl, "Y"=w307:dbl, "good?"=w309:bool)
                          n158 = case shown="True" w309 {
                            selector: w309 -> [w311 w321]
                            tunnel: w308 -> [w313 w327]
                            tunnel: w307 -> [w312 w326]
                            tunnel: w306 -> [_ w325]
                            tunnel: w305 -> [w314 w322]
                            tunnel: w304 -> [_ w324]
                            tunnel: w303 -> [_ w323]
                            tunnel: w301 -> [_ w320]
                            tunnel: w300 -> [_ w319]
                            tunnel: [w314 w318] -> w299
                            tunnel: [w313 w317] -> w298
                            tunnel: [w312 w316] -> w297
                            tunnel: [w311 w315] -> w296
                            frame False {
                            }
                            frame True {
                              n159 = stacked-sequence {
                                tunnel: w327 -> [w332 _ w359 w417]
                                tunnel: w326 -> [w331 _ w358 w416]
                                tunnel: w325 -> [w330 _ _ w412]
                                tunnel: w324 -> [w329 _ w352 _]
                                tunnel: w323 -> [_ w339 w360 _]
                                tunnel: w322 -> [_ _ w361 _]
                                tunnel: w321 -> [_ _ w357 _]
                                tunnel: [_ _ w356 _] -> w318
                                tunnel: [_ _ w355 _] -> w317
                                tunnel: [_ _ w354 _] -> w316
                                tunnel: [_ _ w353 _] -> w315
                                tunnel: w320 -> [_ _ w351 _]
                                tunnel: w319 -> [_ _ w350 _]
                                frame #0 {
                                # "go to tether"
                                n160 = local read "Pixel Calibration"() -> (w335:cluster{"X (nm/px)":dbl, "Y (nm/px)":dbl})
                                n161 = Wait (ms)(milliseconds to wait=w330) -> ()  [unwired: 1 out]
                                n162 = Bundle("X"=w332, "Y"=w331) -> (w338:cluster{"X":dbl, "Y":dbl})  [unwired: 1 in]
                                n163 = Multiply(x=w338, y=w335) -> (x*y=w337:cluster{dbl, dbl})
                                n164 = local write "status:"("moving piezo to target") -> ()
                                n165 = Cluster To Array(cluster=w337) -> (array=w336:dbl[])
                                n166 = Divide(x=w336, y=1000000.0) -> (x/y=w334:dbl[])
                                n167 = shared-variable "My Computer\\SharedVariables.lvlib\\ImageClick"(w334) -> ()  [unwired: 1 in, 1 out]
                                n168 = local write "Last sent value (mm)"(w334) -> ()
                                "#tethers" <- w329
                                }
                                frame #1 {
                                n169 = flat-sequence {
                                tunnel: w339 -> [w342]
                                tunnel: w339 -> [w344]
                                tunnel: w339 -> [w347]
                                frame #0 {
                                n170 = local write "cmd2daq"("check" ("Combo Box")) -> ()
                                n171 = Wait (ms)(milliseconds to wait=w342) -> ()  [unwired: 1 out]
                                }
                                frame #1 {
                                n172 = local write "executed?"(FALSE ("executed?")) -> ()
                                }
                                frame #2 {
                                n173 = while {
                                tunnel: w344 -> [w346]
                                stop <- w345 stop-if-true
                                n174 = local read "executed?"() -> (w345:bool)
                                n175 = Wait (ms)(milliseconds to wait=w346) -> ()  [unwired: 1 out]
                                }
                                }
                                frame #3 {
                                n176 = Wait (ms)(milliseconds to wait=w347) -> ()  [unwired: 1 out]
                                }
                                }
                                n177 = local write "status:"("waiting for check to be finished") -> ()
                                }
                                frame #2 {
                                n178 = local read "result_from_daq"() -> (w348:string)
                                n179 = case shown="\"good tether\"" w348 {
                                tunnel: w361 -> [w365 w372]
                                tunnel: w360 -> [_ w373]
                                tunnel: w359 -> [w364 w369]
                                tunnel: w358 -> [w363 w368]
                                tunnel: w357 -> [_ w371]
                                tunnel: [w365 w372] -> w356
                                tunnel: [w364 w369] -> w355
                                tunnel: [w363 w368] -> w354
                                tunnel: [FALSE w371] -> w353
                                tunnel: w352 -> [_ w370]
                                tunnel: w351 -> [_ w367]
                                tunnel: w350 -> [_ w366]
                                frame "bad tether", Default {
                                # "set the bad tether to bad,\nso in the next loop, do not use it"
                                }
                                frame "good tether" {
                                n180 = stacked-sequence {
                                tunnel: w373 -> [w374 w384 w405]
                                tunnel: w370 -> [_ w400 _]
                                tunnel: w369 -> [_ w398 _]
                                tunnel: w368 -> [_ w397 _]
                                tunnel: w367 -> [_ w391 _]
                                tunnel: w366 -> [_ w387 _]
                                frame #0 {
                                n181 = flat-sequence {
                                tunnel: w374 -> [w375]
                                tunnel: w374 -> [w377]
                                tunnel: w374 -> [w379]
                                tunnel: w374 -> [w382]
                                frame #0 {
                                n182 = Wait (ms)(milliseconds to wait=w375) -> ()  [unwired: 1 out]
                                n183 = local write "cmd2daq"("run" ("Combo Box")) -> ()
                                }
                                frame #1 {
                                n184 = local write "executed?"(FALSE ("executed?")) -> ()
                                n185 = Wait (ms)(milliseconds to wait=w377) -> ()  [unwired: 1 out]
                                }
                                frame #2 {
                                n186 = while {
                                tunnel: w379 -> [w380]
                                stop <- w381 stop-if-true
                                n187 = local read "executed?"() -> (w381:bool)
                                n188 = Wait (ms)(milliseconds to wait=w380) -> ()  [unwired: 1 out]
                                }
                                }
                                frame #3 {
                                n189 = Wait (ms)(milliseconds to wait=w382) -> ()  [unwired: 1 out]
                                }
                                }
                                }
                                frame #1 {
                                w389 = "\r\n"
                                n190 = Wait (ms)(milliseconds to wait=w384) -> ()  [unwired: 1 out]
                                n191 = Format Value(format string="FOV: %04d", value (0)=w387) -> (output string=w386:string)  [unwired: 1 in]
                                n192 = Format Value(format string="tasklist: %04d", value (0)=w391) -> (output string=w390:string)  [unwired: 1 in]
                                n193 = Get Date/Time In Seconds() -> (seconds since 1Jan1904=w404:timestamp)
                                n194 = Get Date/Time String(seconds (now)=w404) -> (date string=w394:string, time string=w393:string)  [unwired: 2 in]
                                n195 = Format Value(format string="%.6f)", value (0)=w397) -> (output string=w395:string)  [unwired: 1 in]
                                n196 = Format Value(format string="tether index: %04d", value (0)=w400) -> (output string=w399:string)  [unwired: 1 in]
                                n197 = Format Value(format string="tether coordinates: (%.6f, ", value (0)=w398) -> (output string=w396:string)  [unwired: 1 in]
                                n198 = Concatenate Strings("descrptn, " ("Combo Box"), w386, w389, w390, w389, w399, w389, w396, w395, w389, w394, w393, w389) -> (w385:string)
                                n199 = local write "cmd2daq"(w385) -> ()
                                }
                                frame #2 {
                                n200 = flat-sequence {
                                tunnel: w405 -> [w406]
                                tunnel: w405 -> [w408]
                                tunnel: w405 -> [w411]
                                frame #0 {
                                n201 = local write "executed?"(FALSE ("executed?")) -> ()
                                n202 = Wait (ms)(milliseconds to wait=w406) -> ()  [unwired: 1 out]
                                }
                                frame #1 {
                                n203 = while {
                                tunnel: w408 -> [w409]
                                stop <- w410 stop-if-true
                                n204 = Wait (ms)(milliseconds to wait=w409) -> ()  [unwired: 1 out]
                                n205 = local read "executed?"() -> (w410:bool)
                                }
                                }
                                frame #2 {
                                n206 = Wait (ms)(milliseconds to wait=w411) -> ()  [unwired: 1 out]
                                }
                                }
                                }
                                }
                                }
                                }
                                n207 = local write "status:"("waiting for tasklist to be finished") -> ()
                                }
                                frame #3 {
                                # "go back to center"
                                n208 = local read "Pixel Calibration"() -> (w421:cluster{"X (nm/px)":dbl, "Y (nm/px)":dbl})
                                n209 = Wait (ms)(milliseconds to wait=w412) -> ()  [unwired: 1 out]
                                n210 = Bundle("X"=w417, "Y"=w416) -> (w415:cluster{"X":dbl, "Y":dbl})  [unwired: 1 in]
                                n211 = Negate(x=w415) -> (-x=w414:cluster{"X":dbl, "Y":dbl})
                                n212 = local write "status:"("moving piezo back to center") -> ()
                                n213 = Multiply(x=w414, y=w421) -> (x*y=w419:cluster{dbl, dbl})
                                n214 = Cluster To Array(cluster=w419) -> (array=w420:dbl[])
                                n215 = Divide(x=w420, y=1000000.0) -> (x/y=w422:dbl[])
                                n216 = shared-variable "My Computer\\SharedVariables.lvlib\\ImageClick"(w422) -> ()  [unwired: 1 in, 1 out]
                                n217 = local write "Last sent value (mm)"(w422) -> ()
                                }
                              }
                            }
                          }
                          n218 = local read "start automatic measurement"() -> (w302:bool)
                          n219 = Bundle("index"=w299, "X"=w298, "Y"=w297, w296) -> (w295:cluster{"index":i32, "X":dbl, "Y":dbl, bool})  [unwired: 1 in]
                        }
                        n220 = local write "information of tethers"(w290) -> ()
                        "#tasklist" <- w292
                      }
                      frame #1 {
                        n221 = local write "status:"("next tasklist..." ("status")) -> ()
                        n222 = local write "cmd2daq"("go to next tasklist" ("Combo Box")) -> ()
                        n223 = Wait (ms)(milliseconds to wait=w424) -> ()  [unwired: 1 out]
                      }
                      frame #2 {
                        n224 = local write "executed?"(FALSE ("executed?")) -> ()
                        n225 = Wait (ms)(milliseconds to wait=w426) -> ()  [unwired: 1 out]
                      }
                      frame #3 {
                        # "tasklist changed"
                        n226 = while {
                          tunnel: w428 -> [w429]
                          stop <- w430 stop-if-true
                          n227 = local read "executed?"() -> (w430:bool)
                          n228 = Wait (ms)(milliseconds to wait=w429) -> ()  [unwired: 1 out]
                        }
                      }
                    }
                    n229 = local read "start automatic measurement"() -> (w288:bool)
                  }
                }
                frame #2 {
                  n230 = Quotient & Remainder(x=w431, y=30) -> (x-y*floor(x/y)=w433:i32)  [unwired: 1 out]
                  n231 = case shown="1.., Default" w433 {
                    tunnel: [w448 -700] -> w435
                    tunnel: [w447 0] -> w434
                    tunnel: w431 -> [w445 _]
                    frame 1.., Default {
                      n232 = Quotient & Remainder(x=w445, y=60) -> (x-y*floor(x/y)=w444:i32)  [unwired: 1 out]
                      n233 = case shown="..99" w444 {
                        tunnel: [0 0] -> w448
                        tunnel: [-700 700] -> w447
                        frame ..99 {
                        }
                        frame 100.. {
                        }
                      }
                    }
                    frame 0 {
                    }
                  }
                  n234 = local write "status:"("moving to the next FOV") -> ()
                  n235 = Wait (ms)(milliseconds to wait=u32 1000) -> ()  [unwired: 1 out]
                  n236 = local read "Pixel Calibration"() -> (w441:cluster{"X (nm/px)":dbl, "Y (nm/px)":dbl})
                  n237 = Bundle(w434, w435) -> (w438:cluster{i32, i32})  [unwired: 1 in]
                  n238 = Multiply(x=w438, y=w441) -> (x*y=w439:cluster{dbl, dbl})
                  n239 = Cluster To Array(cluster=w439) -> (array=w440:dbl[])
                  n240 = Divide(x=w440, y=1000000.0) -> (x/y=w442:dbl[])
                  n241 = shared-variable "My Computer\\SharedVariables.lvlib\\ImageClick"(w442) -> ()  [unwired: 1 in, 1 out]
                  n242 = local write "Last sent value (mm)"(w442) -> ()
                }
              }
              n243 = local read "start automatic measurement"() -> (w218:bool)
            }
          }
        }
        n244 = local write "executed?"(TRUE ("executed?")) -> ()
        n245 = local write "cmd2daq"("" ("cmd2daq")) -> ()
        n246 = local write "result_from_daq"("" ("result_from_daq")) -> ()
      }
      event "stop": Value Change {
        n247 = event-data() -> ()  [unwired: 1 in, 6 out]
      }
    }
  }
  "status:" <- "" ("status:")
